vi "Start TCP.vi"(8 "error in (no error)":errorcluster, 11 "Vecto in":refnum<class "Vecto.lvclass">) -> (0 "error out":errorcluster, 3 "Vecto out":refnum<class "Vecto.lvclass">)   [LabVIEW 2020, in "Vecto.lvlib" / "Vecto.lvclass"]
uses:
  Vecto.lvclass
  Node Config/Node Config.lvclass
  TCPMessaging/TCPMessaging.lvclass
  NodeDiscovery/NodeDiscovery.lvclass
  VectoService/VectoInfo.lvclass
  proto/ServiceType/Enumeration.ctl
  proto/ServiceType/ServiceType.lvlib
  Connection Type.ctl
  Vecto.lvlib
  Connection Info.ctl
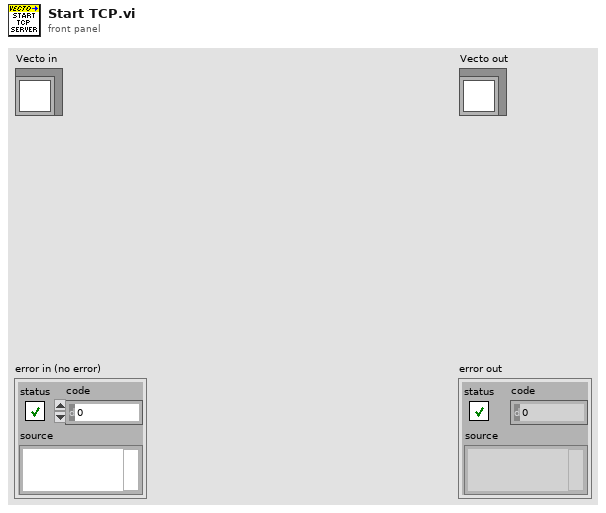
[diagram p1: front panel]
types:
  T1 = typedef "Vecto.lvlib/Connection Type.ctl" = enum16{"TCP", "Telemetry", "Discovery", "HTTP"}
  T2 = typedef "Vecto.lvlib/Connection Info.ctl" = cluster{"Name":string, "Type":T1, "RXCount":i32, "TXCount":i32, "Connected":bool, "RemoteIP":u32, "RemotePort":u16, "LocalPort":u16, "Node ID":u32}
  T3 = typedef "ServiceType.lvlib/Enumeration.ctl" = enum16{"SERVICETYPE_UNKNOWN", "SERVICETYPE_TCPSERVER", "SERVICETYPE_HTTPSERVER"}
  T4 = typedef "Vecto.lvlib/Node Config.lvclass/TCP Messaging Info.ctl" = cluster{"Address":string, "Port":u16, "Server (Client)":bool}
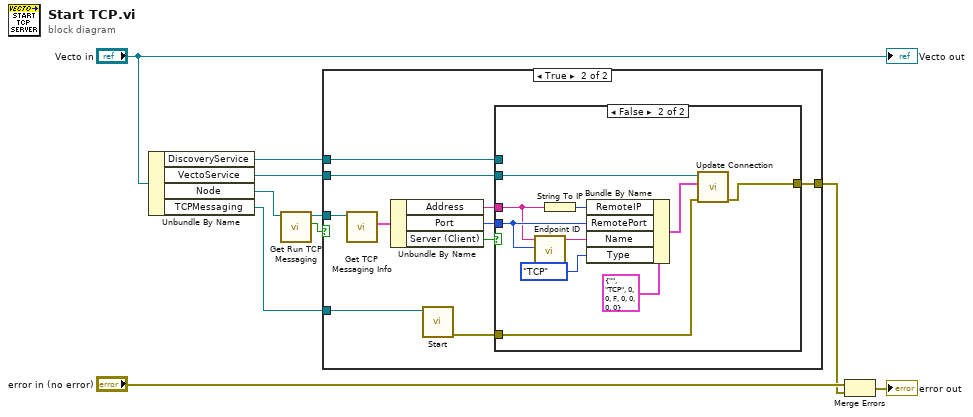
[diagram p0: block diagram]
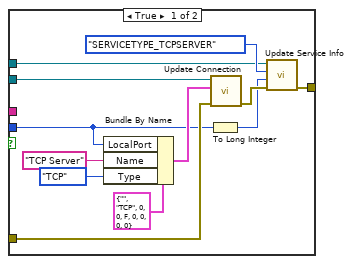
[diagram p3: hidden frame]
diagram:
  n1 = Unbundle By Name("Vecto in") -> ("DiscoveryService"=w4:refnum<class "NodeDiscovery.lvclass">, "VectoService"=w5:refnum<class "VectoInfo.lvclass">, "Node"=w9:refnum<class "Node Config.lvclass">, "TCPMessaging"=w3:refnum<class "TCPMessaging.lvclass">)
  n2 = call "Get Run TCP Messaging.vi"("Node Config in"=w9) -> ("Run TCP Messaging"=w8:bool, "Node Config out"=w2:refnum<class "Node Config.lvclass">)  [unwired: 8 in, 1 out]
  n3 = case shown="True" w8 {
    tunnel: [_ w11] -> w6
    tunnel: w5 -> [_ w17]
    tunnel: w4 -> [_ w16]
    tunnel: w3 -> [_ w20]
    tunnel: w2 -> [_ w19]
    frame False {
    }
    frame True {
      n4 = call "Get TCP Messaging Info.vi"("Node Config in"=w19) -> ("TCP Messaging Info"=w18:T4)  [unwired: 8 in, 2 out]
      n5 = Unbundle By Name(w18) -> ("Address"=w13:string, "Port"=w15:u16, "Server (Client)"=w14:bool)
      n6 = call "Start.vi"("TCPMessaging in"=w20) -> ("error out"=w12:errorcluster)  [unwired: 9 in, 1 out]
      n7 = case shown="False" w14 {
        tunnel: w17 -> [w30 w41]
        tunnel: w16 -> [w28 _]
        tunnel: w15 -> [w22 w34]
        tunnel: w13 -> [_ w33]
        tunnel: w12 -> [w32 w42]
        tunnel: [w21 w37] -> w11
        frame True {
          n8 = Bundle By Name(cluster=T2 {"Name"="", "Type"=enum."TCP", "RXCount"=0, "TXCount"=0, "Connected"=FALSE, "RemoteIP"=0, "RemotePort"=0, "LocalPort"=0, "Node ID"=0} ("Connection Info"), "LocalPort"=w22, "Name"="TCP Server", "Type"=Connection_Type."TCP") -> (w25:T2)
          n9 = To Long Integer(number=w22) -> (32bit integer=w27:i32)
          n10 = call "Update Connection.vi"("error in (no error)"=w32, "Connection Info"=w25, "VectoService in"=w30) -> ("error out"=w31:errorcluster)  [unwired: 7 in, 1 out]
          n11 = call "Update Service Info.vi"("error in (no error)"=w31, "Port"=w27, "Type"=Enumeration."SERVICETYPE_TCPSERVER", "DiscoveryService in"=w28) -> ("error out"=w21:errorcluster)  [unwired: 6 in, 1 out]
        }
        frame False {
          n12 = call "Endpoint ID.vi"("Remote Port"=w34, "Remote Address"=w33) -> ("Endpoint ID"=w35:string)  [unwired: 9 in]
          n13 = String To IP(1:w33) -> (0:w36:u32)
          n14 = Bundle By Name(cluster=T2 {"Name"="", "Type"=enum."TCP", "RXCount"=0, "TXCount"=0, "Connected"=FALSE, "RemoteIP"=0, "RemotePort"=0, "LocalPort"=0, "Node ID"=0} ("Connection Info"), "RemoteIP"=w36, "RemotePort"=w34, "Name"=w35, "Type"=Connection_Type."TCP") -> (w39:T2)
          n15 = call "Update Connection.vi"("error in (no error)"=w42, "Connection Info"=w39, "VectoService in"=w41) -> ("error out"=w37:errorcluster)  [unwired: 7 in, 1 out]
        }
      }
    }
  }
  n16 = Merge Errors("error in (no error)", w6) -> (→"error out":errorcluster)
  "Vecto out" <- "Vecto in"
